vi "axex_vi_tree.vi"   [LabVIEW 2020, in "AX Excel.lvlib"]
uses:
  AX Excel.lvlib
  axex_read_cell.vi
  axex_write_cell.vi
panel:
  # "SEE DIAGRAM\nFOR VI Tree"
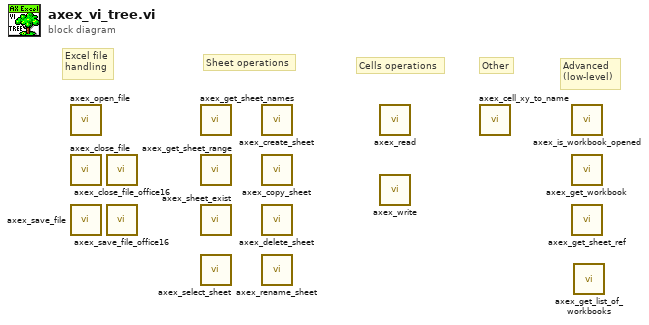
[diagram p0: block diagram]
diagram:
  # "Other"
  # "Advanced\n(low-level)"
  # "Cells operations"
  # "Sheet operations"
  # "Excel file\nhandling"
  n1 = call "axex_open_file.vi"() -> ()  [unwired: 10 in, 2 out]
  n2 = call "axex_close_file.vi"() -> ()  [unwired: 11 in, 1 out]
  n3 = call "axex_save_file.vi"() -> ()  [unwired: 10 in, 2 out]
  n4 = call "axex_close_file_office16.vi"() -> ()  [unwired: 11 in, 1 out]
  n5 = call "axex_save_file_office16.vi"() -> ()  [unwired: 10 in, 2 out]
  n6 = call "axex_get_sheet_names.vi"() -> ()  [unwired: 7 in, 5 out]
  n7 = call "axex_get_sheet_range.vi"() -> ()  [unwired: 8 in, 4 out]
  n8 = call "axex_sheet_exist.vi"() -> ()  [unwired: 6 in, 6 out]
  n9 = call "axex_select_sheet.vi"() -> ()  [unwired: 8 in, 4 out]
  n10 = call "axex_create_sheet.vi"() -> ()  [unwired: 10 in, 2 out]
  n11 = call "axex_copy_sheet.vi"() -> ()  [unwired: 10 in, 2 out]
  n12 = call "axex_delete_sheet.vi"() -> ()  [unwired: 10 in, 2 out]
  n13 = call "axex_rename_sheet.vi"() -> ()  [unwired: 10 in, 2 out]
  n14 = call-poly "axex_read.vi"() -> ()  [unwired: 9 in, 3 out]
  n15 = call-poly "axex_write.vi"() -> ()  [unwired: 10 in, 2 out]
  n16 = call "axex_cell_xy_to_name.vi"() -> ()  [unwired: 2 in, 4 out]
  n17 = call "axex_is_workbook_opened.vi"() -> ()  [unwired: 10 in, 2 out]
  n18 = call "axex_get_workbook.vi"() -> ()  [unwired: 9 in, 3 out]
  n19 = call "axex_get_sheet_ref.vi"() -> ()  [unwired: 8 in, 4 out]
  n20 = call "axex_get_list_of_workbooks.vi"() -> ()  [unwired: 8 in, 4 out]
